vi "Sensors.vi"() -> ()   [LabVIEW 2018]
uses:
  <vilib>/Rock Robotics/SystemInterfaces/i2clib/i2c_bus.ctl
  <vilib>/Rock Robotics/SystemInterfaces/DIO/FPGA_DIOChannel.ctl
  Type Defs/Read Write.ctl
  <vilib>/Rock Robotics/WPI/Counter/WPI_CounterDigitalInputToDigitalSource.vi
panel:
  out "error out":errorcluster
  in  "Invert Direction (False)":bool=TRUE
  out "Discovered Devices":i32[](array[numeric])
  in  "I2C Bus":T1=enum."Invalid"
  in  "Device Address":u8=39
  out "(hi.lo)":u16
  out "Distance":dbl
  out "Direction":bool
  out "Stopped":bool
  # "Invert For Alpha"
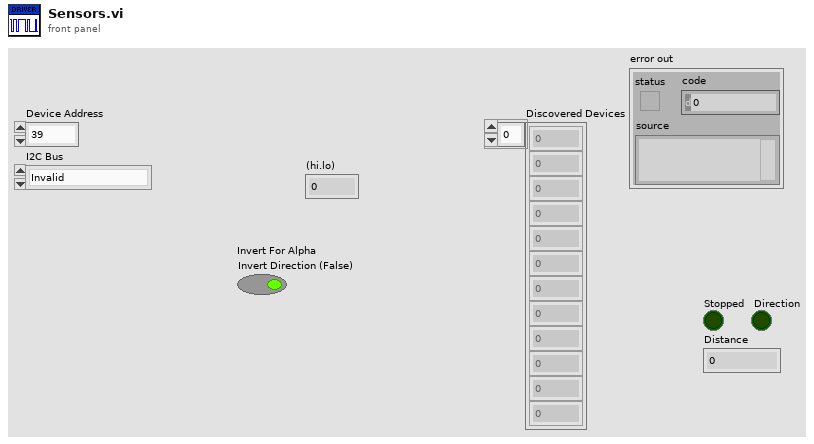
[diagram p1: front panel]
types:
  T1 = typedef "i2c_bus.ctl" = enum16{"I2C On-Board", "I2C MXP", "Invalid"}
  T2 = typedef "FPGA_DIOChannel.ctl" = enum8{"DIO 0", "DIO 1", "DIO 2", "DIO 3", "DIO 4", "DIO 5", "DIO 6", "DIO 7", "DIO 8", "DIO 9", "DIO MXP 0", "DIO MXP 1", "DIO MXP 2", "DIO MXP 3", "DIO MXP 4", "DIO MXP 5", "DIO MXP 6", "DIO MXP 7", "DIO MXP 8", "DIO MXP 9", "DIO MXP 10", "DIO MXP 11", "DIO MXP 12", "DIO MXP 13", "DIO MXP 14", "DIO MXP 15", "SPI Port CS1", "SPI Port CS2", "SPI Port CS3", "SPI Port MISO", "SPI Port MOSI", "Invalid"}
  T3 = typedef "WPI_I2CDevRef.ctl" = cluster{"DevStatus":errorcluster, "Device Address":u8, "Handle":i32, "I2C Bus":T1}
  T4 = typedef "WPI_DigitalInputDevRef.ctl" = cluster{"DevStatus":errorcluster, "DIO Channel":T2}
  T5 = typedef "FPGA_CounterEncoderSourceConvertionLVSourceType.ctl" = cluster{"DevStatus":errorcluster, "AnalogTriggerMode?":bool, "DigitalMode":cluster{"DIO Channel":T6}, "AnalogTriggerMode":cluster{"AnalogTriggerIndex":T7, "OutputType":T8}}
  T6 = typedef "FPGA_DIODigitalSourceChannel.ctl" = enum8{"DIO 0", "DIO 1", "DIO 2", "DIO 3", "DIO 4", "DIO 5", "DIO 6", "DIO 7", "DIO 8", "DIO 9", "DIO MXP 0", "DIO MXP 1", "DIO MXP 2", "DIO MXP 3", "DIO MXP 4", "DIO MXP 5", "DIO MXP 6", "DIO MXP 7", "DIO MXP 8", "DIO MXP 9", "DIO MXP 10", "DIO MXP 11", "DIO MXP 12", "DIO MXP 13", "DIO MXP 14", "DIO MXP 15", "SPI Port CS1", "SPI Port CS2", "SPI Port CS3", "SPI Port MISO", "SPI Port MOSI", "Disabled"}
  T7 = typedef "FPGA_AnalogTriggerIndex.ctl" = enum8{"Trig 0", "Trig 1", "Trig 2", "Trig 3", "Trig 4", "Trig 5", "Trig 6", "Trig 7", "Invalid"}
  T8 = typedef "FPGA_AnalogTriggerOutType.ctl" = enum16{"InWindow", "TriggerState", "Rising", "Falling"}
  T9 = typedef "WPI_EncoderDevRef.ctl" = cluster{"DevStatus":errorcluster, "EncoderIndex":T10, "CounterIndex":T11, "DistancePerCount":dbl, "Decoding Type":T12}
  T10 = typedef "FPGA_EncoderIdx.ctl" = enum8{"Enc 0", "Enc 1", "Enc 2", "Enc 3", "Enc 4", "Enc 5", "Enc 6", "Enc 7", "Invalid"}
  T11 = typedef "FPGA_CounterCtrSystemIndex.ctl" = enum8{"Ctr 0", "Ctr 1", "Ctr 2", "Ctr 3", "Ctr 4", "Ctr 5", "Ctr 6", "Ctr 7", "Invalid"}
  T12 = typedef "WPI_EncoderType.ctl" = enum16{"1x", "2x", "4x"}
  T13 = typedef "Read Write.ctl" = enum16{"Read", "Write"}
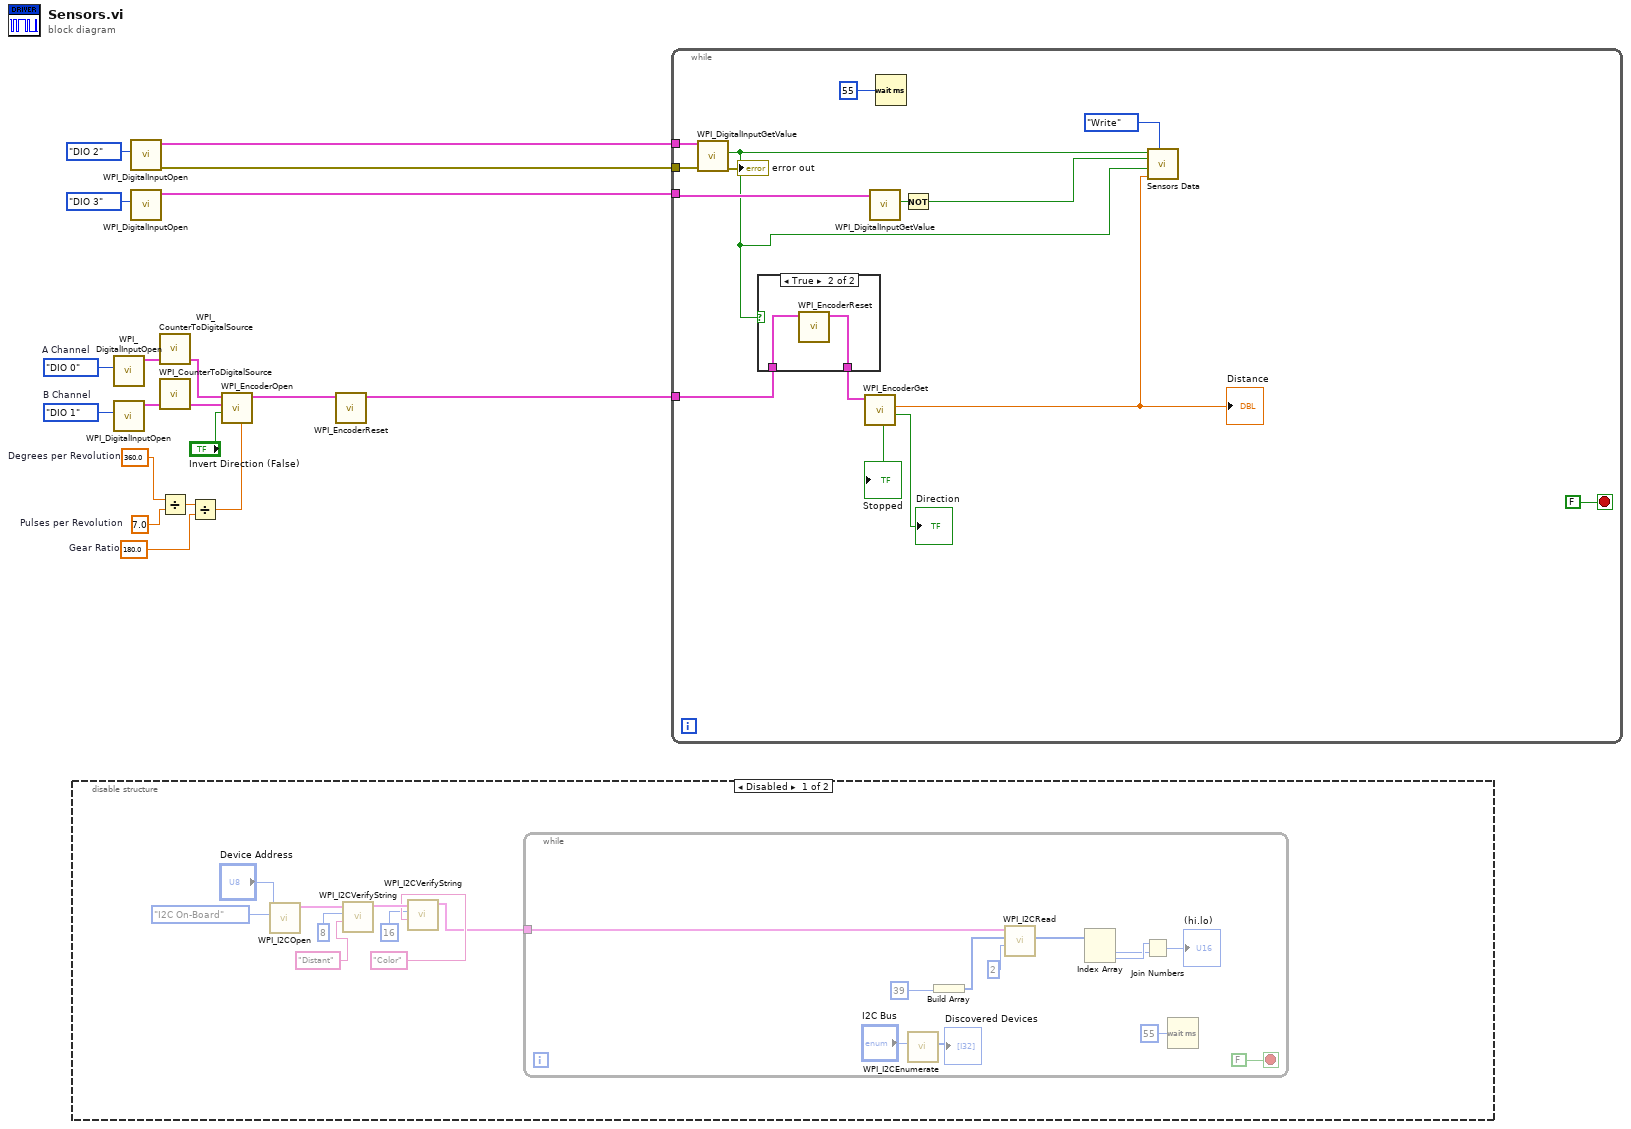
[diagram p0: block diagram]
diagram:
  w6 = 180.0  # Gear Ratio
  w8 = 7.0  # Pulses per Revolution
  w9 = 360.0  # Degrees per Revolution
  w15 = FPGA_DIOChannel."DIO 1"  # B Channel
  w14 = FPGA_DIOChannel."DIO 0"  # A Channel
  n1 = disable-structure shown="Disabled" {
    frame Disabled {
      n2 = call <vilib>:"WPI_I2COpen.vi"("Device Address"="Device Address", "I2C Bus"=i2c_bus."I2C On-Board") -> ("I2CDevRef"=w28:T3)  [unwired: 8 in, 1 out]
      n3 = call <vilib>:"WPI_I2CVerifyString.vi"("Expected"="Distant", "Register Address"=u8 8, "I2CDevRef"=w28) -> ("I2CDevRef"=w27:T3)  [unwired: 7 in, 1 out]
      n4 = call <vilib>:"WPI_I2CVerifyString.vi"("Expected"="Color", "Register Address"=u8 16, "I2CDevRef"=w27) -> ("I2CDevRef"=w20:T3)  [unwired: 7 in, 1 out]
      n5 = while {
        tunnel: w20 -> [w29]
        stop <- FALSE stop-if-true
        n6 = call <vilib>:"WPI_I2CEnumerate.vi"("I2C Bus"="I2C Bus") -> ("Discovered Devices"=→"Discovered Devices":i32[])  [unwired: 10 in]
        n7 = Build Array(u8 39 ("Device Address")) -> (w39:u8[])
        n8 = call <vilib>:"WPI_I2CRead.vi"("I2CBytesToRead"=u8 2, "I2CRegister"=w39, "I2CDevRef"=w29) -> ("Data Out"=w37:u8[])  [unwired: 6 in, 2 out]
        n9 = Index Array(array=w37) -> (element #1=w35:u8, element #2=w36:u8)  [unwired: 2 in]
        n10 = Join Numbers(hi=w36, lo=w35) -> ((hi.lo)=→"(hi.lo)":u16)
        n11 = Wait (ms)(milliseconds to wait=u32 55) -> ()  [unwired: 1 out]
      }
    }
    frame Enabled {
    }
  }
  n12 = call <vilib>:"WPI_DigitalInputOpen.vi"("DIO Channel"=w14) -> ("DigitalInputDevRef"=w11:T4)  [unwired: 1 in, 9 out]
  n13 = call <vilib>:"WPI_DigitalInputOpen.vi"("DIO Channel"=w15) -> ("DigitalInputDevRef"=w12:T4)  [unwired: 1 in, 9 out]
  n14 = call <vilib>:"WPI_DigitalInputOpen.vi"("DIO Channel"=FPGA_DIOChannel."DIO 2") -> ("error out"=w1:errorcluster, "DigitalInputDevRef"=w17:T4)  [unwired: 9 in]
  n15 = call <vilib>:"WPI_DigitalInputOpen.vi"("DIO Channel"=FPGA_DIOChannel."DIO 3") -> ("DigitalInputDevRef"=w16:T4)  [unwired: 9 in, 1 out]
  n16 = call-poly <vilib>:"WPI_CounterToDigitalSource.vi"("DigitalInputDevRef"=w11) -> ("Digital Source"=w10:T5)  [unwired: 6 out]
  n17 = call-poly <vilib>:"WPI_CounterToDigitalSource.vi"("DigitalInputDevRef"=w12) -> ("Digital Source"=w13:T5)  [unwired: 6 out]
  n18 = Divide(x=w9, y=w8) -> (x/y=w7:dbl)
  n19 = Divide(x=w7, y=w6) -> (x/y=w5:dbl)
  n20 = call <vilib>:"WPI_EncoderOpen.vi"("DistancePerCount"=w5, "Invert Direction (False)"="Invert Direction (False)", "BSource"=w13, "ASource"=w10) -> ("EncoderDevRef"=w3:T9)  [unwired: 4 in, 3 out]
  n21 = call <vilib>:"WPI_EncoderReset.vi"("EncoderDevRef"=w3) -> ("EncoderDevRef"=w2:T9)  [unwired: 9 in, 1 out]
  n22 = while {
    tunnel: w17 -> [w53]
    tunnel: w16 -> [w52]
    tunnel: w2 -> [w48]
    tunnel: w1 -> [w45]
    stop <- FALSE stop-if-true
    n23 = call <vilib>:"WPI_DigitalInputGetValue.vi"("error in (no error)"=w45, "DigitalInputDevRef"=w53) -> ("error out"=→"error out":errorcluster, "Value"=w41:bool)  [unwired: 7 in, 1 out]
    n24 = case shown="True" w41 {
      tunnel: w48 -> [w56 w58]
      tunnel: [w56 w57] -> w47
      frame False {
      }
      frame True {
        n25 = call <vilib>:"WPI_EncoderReset.vi"("EncoderDevRef"=w58) -> ("EncoderDevRef"=w57:T9)  [unwired: 9 in, 1 out]
      }
    }
    n26 = call <vilib>:"WPI_EncoderGet.vi"("EncoderDevRef"=w47) -> ("Direction"=→"Direction":bool, "Distance"=w42:dbl, "Stopped"=→"Stopped":bool)  [unwired: 5 in, 3 out]
    "Distance" <- w42
    n27 = call <vilib>:"WPI_DigitalInputGetValue.vi"("DigitalInputDevRef"=w52) -> ("Value"=w46:bool)  [unwired: 8 in, 2 out]
    n28 = Wait (ms)(milliseconds to wait=u32 55 ("millisecond timer value")) -> ()  [unwired: 1 out]
    n29 = Not(x=w46) -> (.not. x?=w43:bool)
    n30 = call "Sensors Data.vi"("Read//Write"=Read_Write."Write", "Distance In"=w42, "Switch Hit?"=w41, "Limit Down In"=w43, "Limit Up In"=w41) -> ()  [unwired: 3 in, 4 out]
  }
